vi "Get Desired Positon.vi"(8 "error in (no error)":errorcluster, 10 "Axis Name":string, 11 "SIM Motion Controller in":refnum<class "SIM Motion Controller.lvclass">) -> (0 "error out":errorcluster, 2 "Raw Current Position":dbl, 3 "SIM Motion Controller out":refnum<class "SIM Motion Controller.lvclass">)   [LabVIEW 2022 SP3, in "SIM Motion Controller.lvclass"]
uses:
  SIM Motion Controller.lvclass
  SIM Motion Controller.lvclass/SIM Motion Controller.ctl
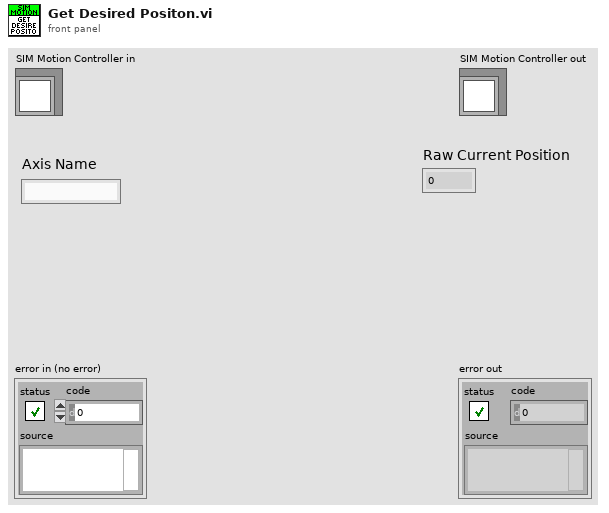
[diagram p1: front panel]
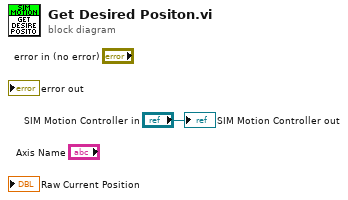
[diagram p0: block diagram]
diagram:
  "SIM Motion Controller out" <- "SIM Motion Controller in"
